vi "LoadPixelCoordinates.vi"(0 "spotsize (radius pixel)":u16) -> ()   [LabVIEW 2009]
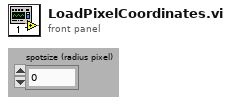
[diagram p1: front panel]
types:
  T1 = enum16{"read/write", "read-only", "write-only", "write-only (truncate)"}
  T2 = cluster{"x0":i32, "y0":i32, "x1":i32, "y1":i32, "ovl std":i32[][]}
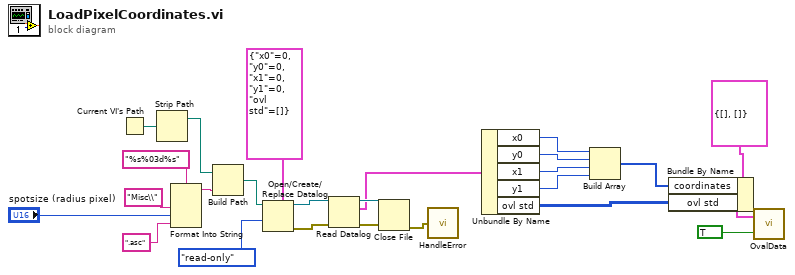
[diagram p0: block diagram]
diagram:
  n1 = Current VI's Path() -> (path=w12:path)
  n2 = Strip Path(path=w12) -> (stripped path=w11:path)  [unwired: 1 out]
  n3 = Format Into String(format string="%s%03d%s", "Misc\\" ("input 1"), "spotsize (radius pixel)", ".asc" ("input 3")) -> (resulting string=w10:string)  [unwired: 2 in, 1 out]
  n4 = Build Path(base path=w11, name or relative path=w10) -> (appended path=w9:path)
  n5 = Open/Create/Replace Datalog(5:T2 {"x0"=0, "y0"=0, "x1"=0, "y1"=0, "ovl std"=[]} ("cluster"), 9:T1."read-only" ("open mode (0)"), 11:w9) -> (0:w8:errorcluster, 3:w6:refnum<k1>)  [unwired: 3 in, 1 out]
  n6 = Read Datalog(4:w8, 7:w6) -> (0:w7:errorcluster, 2:w2:T2, 3:w5:refnum<k1>)  [unwired: 1 in]
  n7 = Close File(refnum=w5, error in=w7) -> (error out=w1:errorcluster)  [unwired: 1 out]
  n8 = call "HandleError.vi"("error in (no error)"=w1) -> ()
  n9 = Unbundle By Name(w2) -> ("x0"=w19:i32, "y0"=w20:i32, "x1"=w21:i32, "y1"=w22:i32, "ovl std"=w23:i32[][])
  n10 = Build Array(w19, w20, w21, w22) -> (w24:i32[])
  n11 = Bundle By Name(cluster=cluster{"coordinates":i32[], "ovl std":i32[][]} {"coordinates"=[], "ovl std"=[]} ("data"), "coordinates"=w24, "ovl std"=w23) -> (w17:cluster{"coordinates":i32[], "ovl std":i32[][]})
  n12 = call "OvalData.vi"("changed?"=TRUE, "data 2"=w17) -> ()  [unwired: 1 out]
